vi "pr650_writecommand.vi"(0 "error in":errorcluster, 1 "write buffer":string="B1", 2 "VISA resource name in":refnum<visa-resource-name>) -> (3 "error out":errorcluster, 4 "return count":u32, 6 "VISA resource name out":refnum<visa-resource-name>)   [LabVIEW 2010]
uses:
  <vilib>/Instr/_visa.llb/VISA Flush IO Buffer Mask.ctl
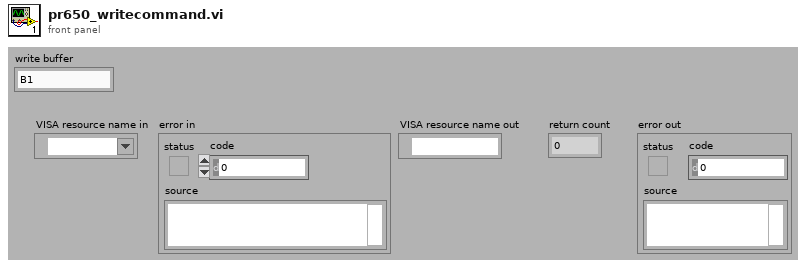
[diagram p1: front panel]
types:
  T1 = typedef "VISA Flush IO Buffer Mask.ctl" = u16
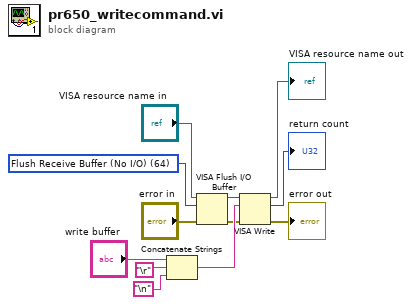
[diagram p0: block diagram]
diagram:
  w1 = T1 64 items=["Flush Receive Buffer"=16, "Write Transmit Buffer to Device"=32, "Flush Receive Buffer (No I/O)"=64, "Flush Transmit Buffer"=128] ("Mask")
  n1 = Concatenate Strings("write buffer", "\r", "\n") -> (w12:string)
  n2 = VISA Flush I/O Buffer(VISA resource name="VISA resource name in", mask (16)=w1, error in (no error)="error in") -> (VISA resource name out=w4:refnum<visa-resource-name>, error out=w2:errorcluster)
  n3 = VISA Write(VISA resource name=w4, write buffer=w12, error in (no error)=w2) -> (VISA resource name out=→"VISA resource name out":refnum<visa-resource-name>, return count=→"return count":u32, error out=→"error out":errorcluster)
